vi "Unset Run Icon Editor from Source.vi"   [LabVIEW 2020]
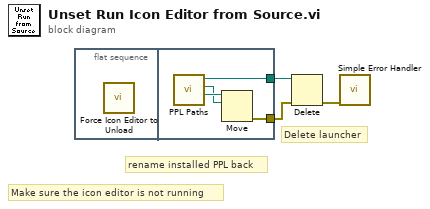
[diagram p0: block diagram]
diagram:
  # "Delete launcher"
  # "rename installed PPL back"
  # "Make sure the icon editor is not running"
  n1 = flat-sequence {
    tunnel: [w7] -> w3
    tunnel: [w4] -> w1
    frame #0 {
      n2 = call "Force Icon Editor to Unload.vi"() -> ()  [unwired: 12 in]
    }
    frame #1 {
      n3 = call "PPL Paths.vi"() -> ("Renamed PPL Path"=w6:path, "PPL Path"=w5:path, "lv_icon Path"=w4:path)  [unwired: 9 in]
      n4 = Move(source path=w6, 10:w5) -> (error out=w7:errorcluster)  [unwired: 3 in, 2 out]
    }
  }
  n5 = Delete(path (use dialog)=w1, error in=w3) -> (error out=w2:errorcluster)  [unwired: 3 in, 2 out]
  n6 = call <vilib>:"Simple Error Handler.vi"("error in (no error)"=w2) -> ()  [unwired: 4 in, 5 out]
